vi "Find Window_KT.vi"(11 "Window Title":string) -> (3 "hWnd":u32)   [LabVIEW 2017, in "KTools.lvlib"]
doc: "<-----------Find Window------------>\nReturns handle for the given window title."
uses:
  KTools.lvlib
  user32.dll
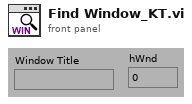
[diagram p1: front panel]
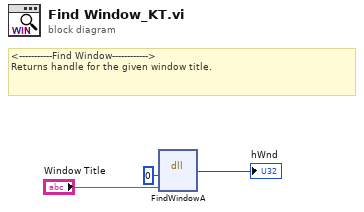
[diagram p0: block diagram]
diagram:
  # "<-----------Find Window------------>\nReturns handle for the given window title."
  n1 = dll-call lib="user32.dll" fn="FindWindowA"("lpszClassName"=u32 0, "lpszWindowName"="Window Title") -> ("hWnd"=→"hWnd":u32)  [unwired: 5 in, 2 out]
